vi "FPGA_2R_ADC_W_DAC.vi"() -> ()   [LabVIEW 2019]
uses:
  <vilib>/rvi/Emulation/niFpgaGetClockAttributes.vi
  <vilib>/rvi/Emulation/niFpgaSctlEmulationGetInTimedLoop.vi
  <vilib>/rvi/Emulation/niFpgaEmulationReportErrorSimple.vi
  <vilib>/rvi/eio/common/nirviEmuTemplateMethod_errors.vi
  <vilib>/rvi/Emulation/niFpgaCriticalErrorInLSC.vi
  <vilib>/eio/EIONode/EIONode.xnode
panel:
  in  "Count(Ticks)":u32=800
  out "ADC Read":bool[](array[boolean])
  in  "stop 2":bool
  out "Data array":bool[](array[boolean])
  out "Encoder B Ref":bool
  out "Encoder A Ref":bool
  out "Encoder B":i32(graph)
  out "Encoder A":i32
  in  "ENC stop":bool
  in  "DAC 3 write":bool[](array[boolean])=[FALSE, FALSE, FALSE, FALSE, FALSE, FALSE, FALSE, FALSE, FALSE, FALSE, FALSE, FALSE, FALSE, FALSE, FALSE, FALSE]
  in  "DAC 2 write":bool[](array[boolean])=[FALSE, FALSE, FALSE, FALSE, FALSE, FALSE, FALSE, FALSE, FALSE, FALSE, FALSE, FALSE, FALSE, FALSE, FALSE, FALSE]
  in  "DAC 1 write":bool[](array[boolean])=[FALSE, FALSE, FALSE, FALSE, FALSE, FALSE, FALSE, FALSE, FALSE, FALSE, FALSE, FALSE, FALSE, FALSE, FALSE, FALSE]
  in  "DAQ stop":bool
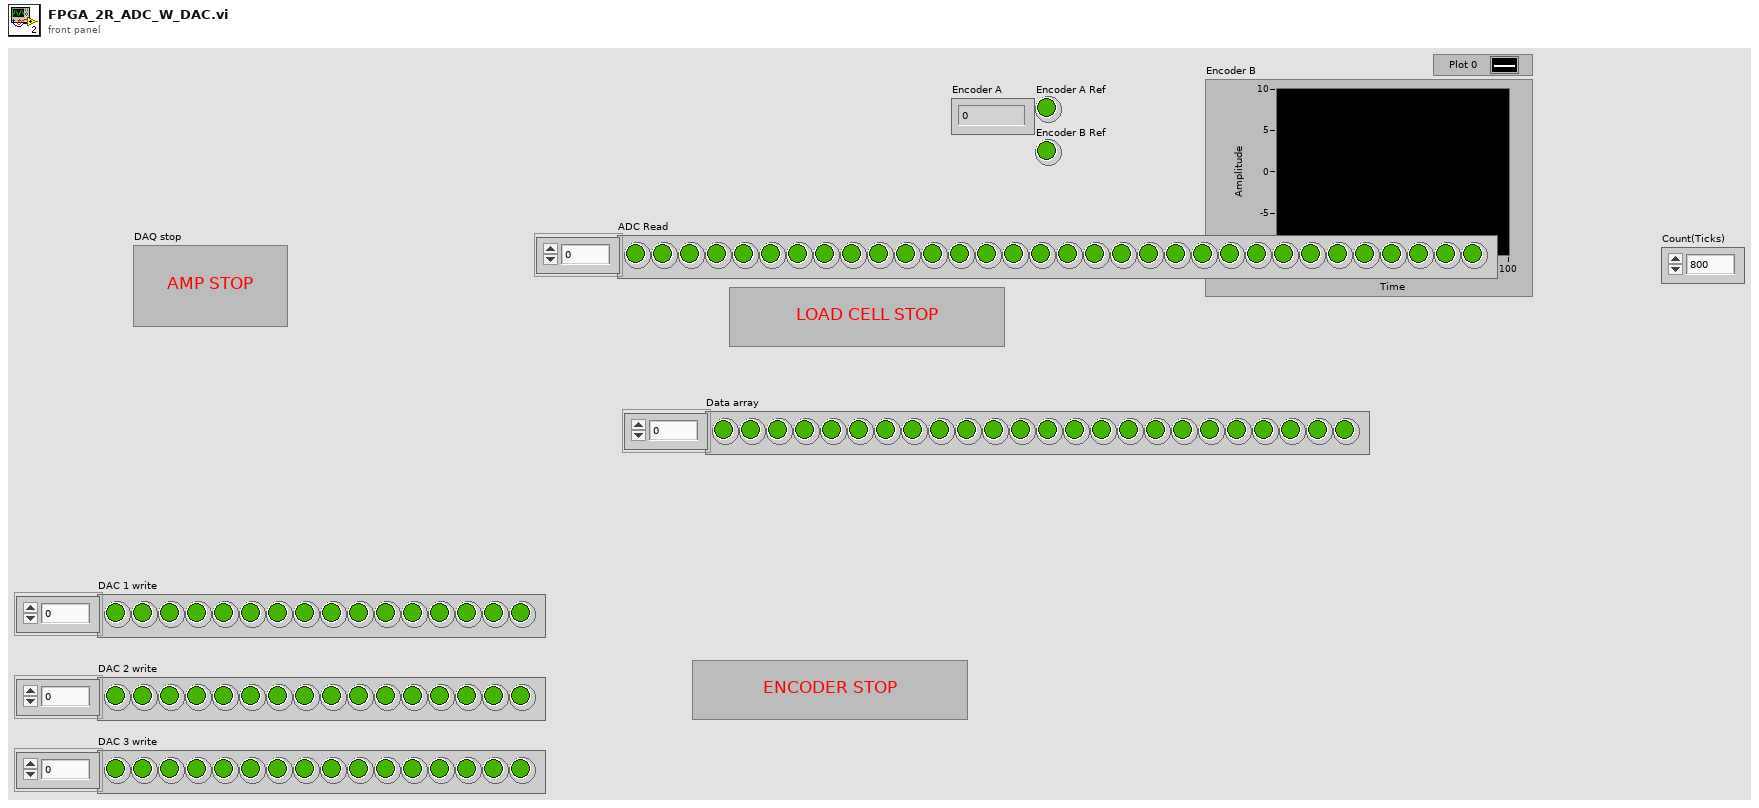
[diagram p1: front panel]
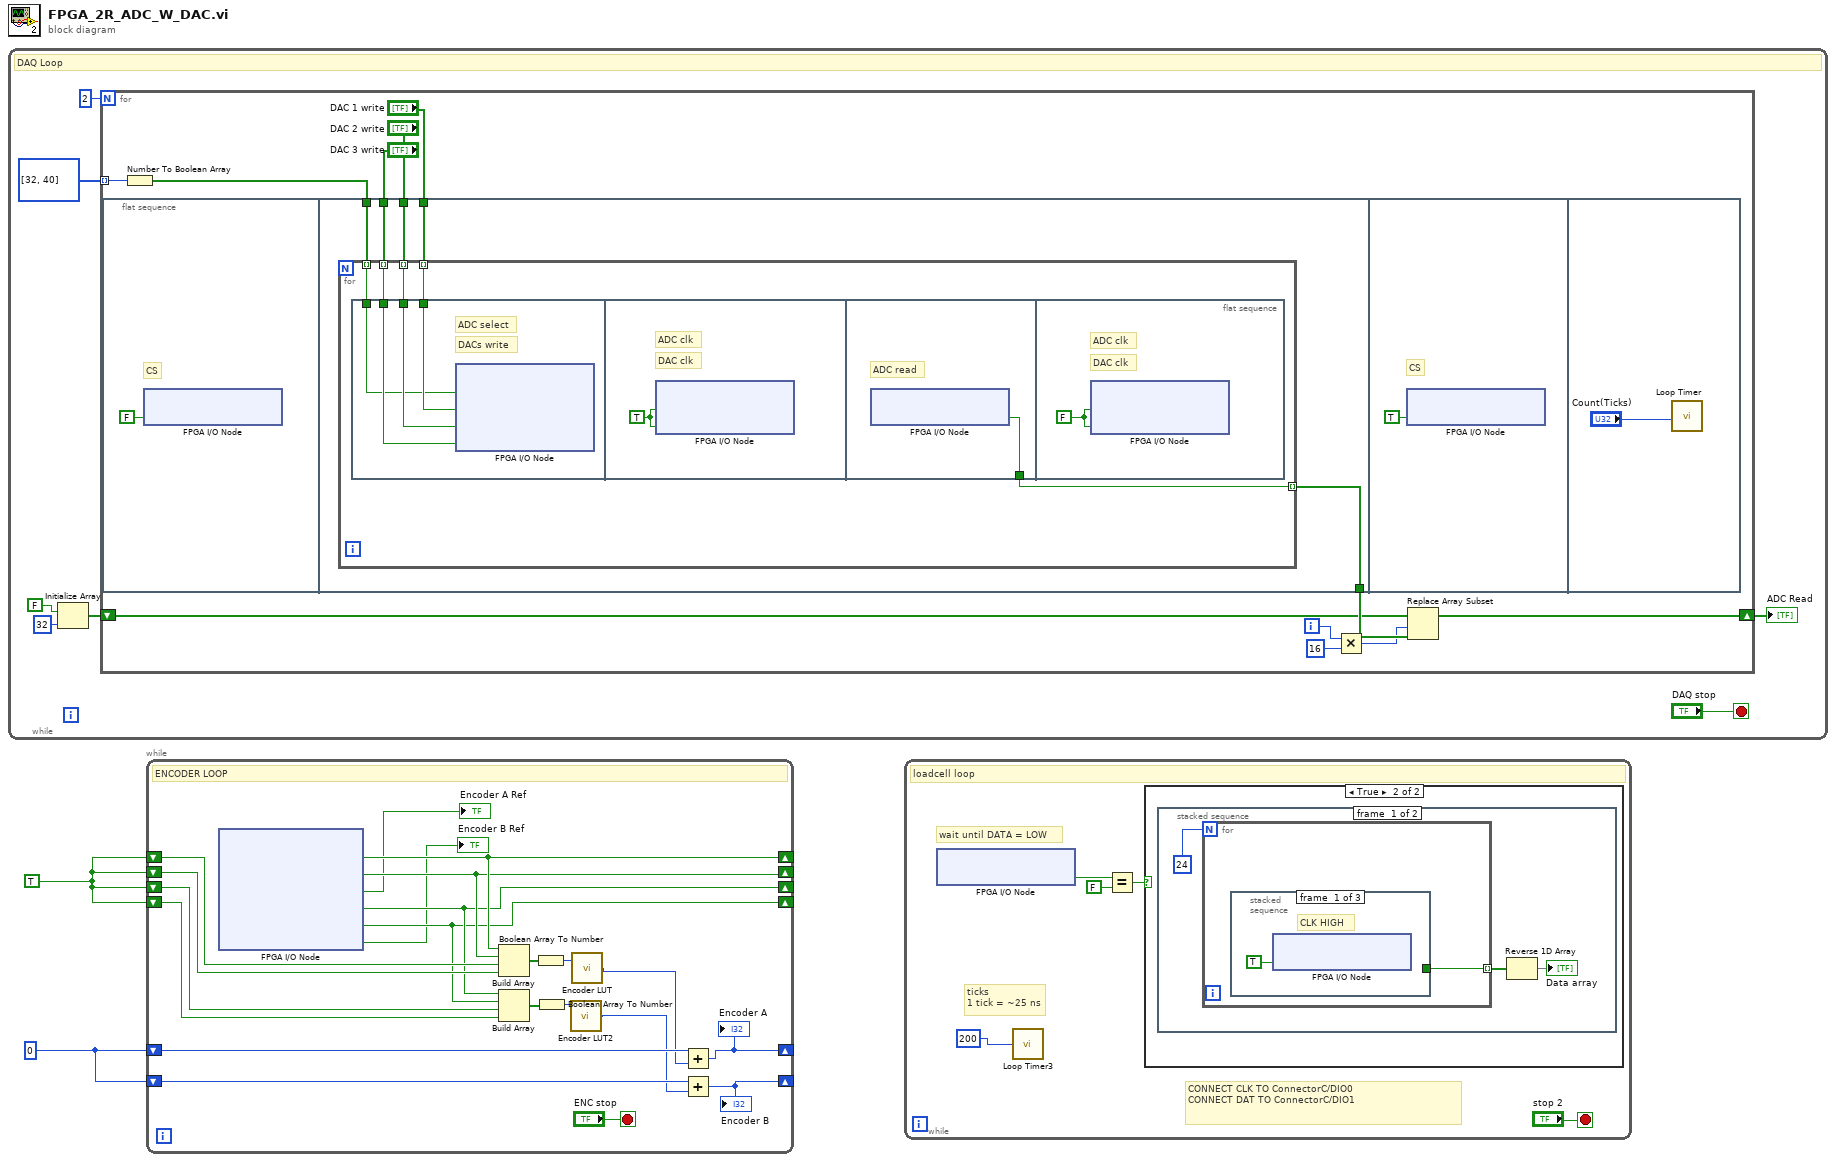
[diagram p0: block diagram]
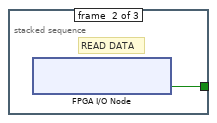
[diagram p3: hidden frame]
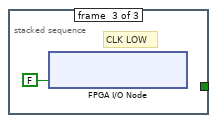
[diagram p4: hidden frame]
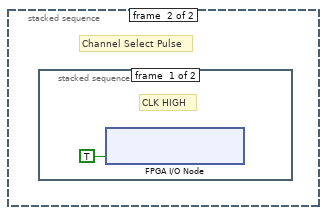
[diagram p5: hidden frame]
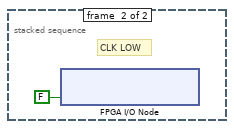
[diagram p6: hidden frame]
diagram:
  w1 = TRUE
  w2 = 0
  n1 = while {
    stop <- "DAQ stop" stop-if-true
    # "DAQ Loop"
    n2 = Initialize Array(FALSE, 32 ("dimension size")) -> (w5:bool[])
    n3 = for {
      N: 2 -> [_]
      shift-right: [w10] -> w3
      shift-left: w5 -> [w12]
      tunnel: u16[] [32, 40] -> [w11] mode=indexing
      i -> [w16]
      n4 = flat-sequence {
        tunnel: "DAC 1 write" -> [w26]
        tunnel: "DAC 2 write" -> [w25]
        tunnel: "DAC 3 write" -> [w24]
        tunnel: w17 -> [w23]
        tunnel: [w22] -> w14
        frame #0 {
          # "CS"
          n5 = xnode "FPGA I/O Node"("ConnectorA/DIO4"=FALSE) -> ()  [unwired: 1 in, 1 out]
        }
        frame #1 {
          n6 = for {
            tunnel: w26 -> [w31] mode=indexing
            tunnel: w25 -> [w30] mode=indexing
            tunnel: w24 -> [w29] mode=indexing
            tunnel: [w28] -> w22 mode=indexing
            tunnel: w23 -> [w27] mode=indexing
            n7 = flat-sequence {
              tunnel: w31 -> [w33]
              tunnel: w30 -> [w35]
              tunnel: w29 -> [w34]
              tunnel: w27 -> [w32]
              tunnel: [w37] -> w28
              frame #0 {
                # "DACs write"
                # "ADC select"
                n8 = xnode "FPGA I/O Node"("ConnectorA/DIO2"=w32, "ConnectorA/DIO6"=w33, "ConnectorA/DIO7"=w35, "ConnectorA/DIO8"=w34) -> ()  [unwired: 4 in, 4 out]
              }
              frame #1 {
                w36 = TRUE ("ConnectorA/DIO3")
                # "DAC clk"
                # "ADC clk"
                n9 = xnode "FPGA I/O Node"("ConnectorA/DIO3"=w36, "ConnectorA/DIO5"=w36) -> ()  [unwired: 2 in, 2 out]
              }
              frame #2 {
                # "ADC read"
                n10 = xnode "FPGA I/O Node"() -> ("ConnectorA/DIO1"=w37:bool)  [unwired: 1 in, 1 out]
              }
              frame #3 {
                w38 = FALSE ("ConnectorA/DIO3")
                # "DAC clk"
                # "ADC clk"
                n11 = xnode "FPGA I/O Node"("ConnectorA/DIO3"=w38, "ConnectorA/DIO5"=w38) -> ()  [unwired: 2 in, 2 out]
              }
            }
          }
        }
        frame #2 {
          # "CS"
          n12 = xnode "FPGA I/O Node"("ConnectorA/DIO4"=TRUE) -> ()  [unwired: 1 in, 1 out]
        }
        frame #3 {
          n13 = call "Loop Timer"("Count(Ticks)"="Count(Ticks)") -> ()  [unwired: 1 out]
        }
      }
      n14 = Number To Boolean Array(number=w11) -> (Boolean array=w17:bool[])
      n15 = Multiply(x=w16, y=16) -> (x*y=w13:i32)
      n16 = Replace Array Subset(array=w12, new element=w14, index=w13) -> (w10:bool[])
    }
    "ADC Read" <- w3
  }
  n17 = while {
    shift-right: [w46] -> _
    shift-left: w2 -> [w49]
    shift-right: [w54] -> _
    shift-left: w1 -> [w60]
    shift-right: [w53] -> _
    shift-left: w1 -> [w57]
    shift-right: [w52] -> _
    shift-left: w1 -> [w56]
    shift-right: [w51] -> _
    shift-left: w1 -> [w55]
    shift-right: [w47] -> _
    shift-left: w2 -> [w48]
    stop <- "ENC stop" stop-if-true
    # "ENCODER LOOP"
    n18 = xnode "FPGA I/O Node"() -> ("ConnectorA/DIO9"=w54:bool, "ConnectorA/DIO10"=w53:bool, "ConnectorA/DIO11"=→"Encoder A Ref":bool, "ConnectorA/DIO13"=w52:bool, "ConnectorA/DIO14"=w51:bool, "ConnectorA/DIO12"=→"Encoder B Ref":bool)  [unwired: 6 in, 6 out]
    n19 = Build Array(w54, w53, w60, w57) -> (w58:bool[])
    n20 = Build Array(w52, w51, w56, w55) -> (w59:bool[])
    n21 = Boolean Array To Number(Boolean array=w58) -> (number=w43:u8)
    n22 = Boolean Array To Number(Boolean array=w59) -> (number=w42:u8)
    n23 = call "Encoder LUT2"("address"=w42) -> ("data out"=w41:i32)  [unwired: 8 in]
    n24 = call "Encoder LUT"("address"=w43) -> ("data out"=w44:i32)  [unwired: 8 in]
    n25 = Add(x=w49, y=w44) -> (x+y=w46:i32)
    "Encoder A" <- w46
    n26 = Add(x=w48, y=w41) -> (x+y=w47:i32)
    "Encoder B" <- w47
  }
  n27 = while {
    stop <- "stop 2" stop-if-true
    # "CONNECT CLK TO ConnectorC/DIO0\nCONNECT DAT TO ConnectorC/DIO1"
    # "ticks\n1 tick = ~25 ns"
    # "wait until DATA = LOW"
    # "loadcell loop"
    n28 = xnode "FPGA I/O Node"() -> ("ConnectorC/DIO1"=w65:bool)  [unwired: 1 in, 1 out]
    n29 = call "Loop Timer3"("Count(Ticks)"=u32 200) -> ()  [unwired: 1 out]
    n30 = Equal?(x=w65, y=FALSE) -> (x = y?=w63:bool)
    n31 = case shown="True" w63 {
      frame False {
      }
      frame True {
        n32 = stacked-sequence {
          frame #0 {
            n33 = for {
              N: 24 -> [_]
              tunnel: [w70] -> w68 mode=indexing
              n34 = stacked-sequence {
                tunnel: [_ w72 _] -> w70
                frame #0 {
                  # "CLK HIGH"
                  n35 = xnode "FPGA I/O Node"("ConnectorC/DIO0"=TRUE ("ConnectorB/DIO0")) -> ()  [unwired: 1 in, 1 out]
                }
                frame #1 {
                  # "READ DATA"
                  n36 = xnode "FPGA I/O Node"() -> ("ConnectorC/DIO1"=w72:bool)  [unwired: 1 in, 1 out]
                }
                frame #2 {
                  # "CLK LOW"
                  n37 = xnode "FPGA I/O Node"("ConnectorC/DIO0"=FALSE ("ConnectorB/DIO0")) -> ()  [unwired: 1 in, 1 out]
                }
              }
            }
            n38 = Reverse 1D Array(array=w68) -> (reversed array=→"Data array":bool[])
          }
          frame #1 {
            # "Channel Select Pulse"
            n39 = stacked-sequence {
              frame #0 {
                # "CLK HIGH"
                n40 = xnode "FPGA I/O Node"("ConnectorC/DIO0"=TRUE ("ConnectorB/DIO0")) -> ()  [unwired: 1 in, 1 out]
              }
              frame #1 {
                # "CLK LOW"
                n41 = xnode "FPGA I/O Node"("ConnectorC/DIO0"=FALSE ("ConnectorB/DIO0")) -> ()  [unwired: 1 in, 1 out]
              }
            }
          }
        }
      }
    }
  }
